vi "Add Ports Section.vi"(8 "error in":errorcluster, 11 "custom device ref":T1 format="%.0x") -> (0 "error out":errorcluster, 2 "ports ref":T1 format="%.0x", 3 "custom device ref out":T1 format="%.0x")   [LabVIEW 2020, in "ARINC 429 Scripting.lvlib"]
uses:
  ARINC 429 Scripting.lvlib
  <vilib>/NI VeriStand/Custom Device API/Custom Device Item Ref.ctl
  Ballard/Constants.vi
  <vilib>/NI VeriStand/Custom Device API/Custom Device API.lvlib
  Ballard/Ballard ARINC 429 Scripting.lvlib
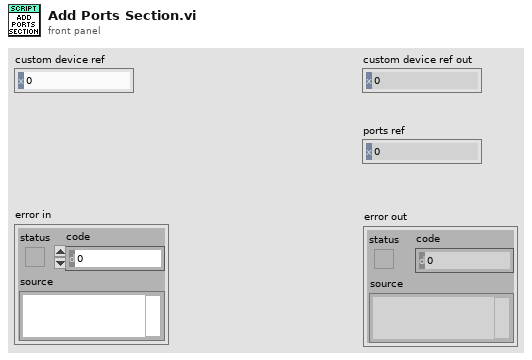
[diagram p1: front panel]
types:
  T1 = typedef "Custom Device API.lvlib/Custom Device Item Ref.ctl" = u64
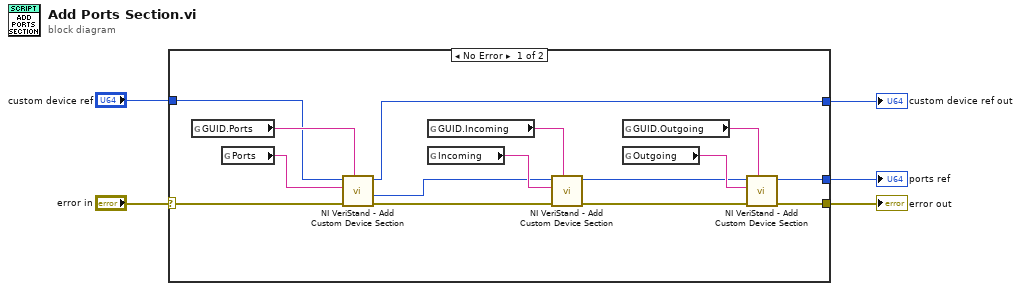
[diagram p0: block diagram]
diagram:
  n1 = case shown="No Error" "error in" {
    selector: "error in" -> [w18 w22]
    tunnel: "custom device ref" -> [w19 w21]
    tunnel: [w8 w22] -> w4
    tunnel: [w17 w21] -> w3
    tunnel: [w6 _] -> w1
    frame No Error {
      n2 = global read "Constants.vi" "GUID.Ports"() -> (w20:string)
      n3 = global read "Constants.vi" "Ports"() -> (w16:string)
      n4 = call <vilib>:"NI VeriStand - Add Custom Device Section.vi"("GUID (Default Section)"=w20, "error in (no error)"=w18, "Section Name"=w16, "Parent Ref in"=w19) -> ("error out"=w13:errorcluster, "Section Ptr"=w12:T1, "Parent Ref out"=w17:T1)  [unwired: 4 in, 1 out]
      n5 = global read "Constants.vi" "GUID.Incoming"() -> (w14:string)
      n6 = global read "Constants.vi" "Incoming"() -> (w15:string)
      n7 = call <vilib>:"NI VeriStand - Add Custom Device Section.vi"("GUID (Default Section)"=w14, "error in (no error)"=w13, "Section Name"=w15, "Parent Ref in"=w12) -> ("error out"=w9:errorcluster, "Parent Ref out"=w7:T1)  [unwired: 4 in, 2 out]
      n8 = global read "Constants.vi" "GUID.Outgoing"() -> (w10:string)
      n9 = global read "Constants.vi" "Outgoing"() -> (w11:string)
      n10 = call <vilib>:"NI VeriStand - Add Custom Device Section.vi"("GUID (Default Section)"=w10, "error in (no error)"=w9, "Section Name"=w11, "Parent Ref in"=w7) -> ("error out"=w8:errorcluster, "Parent Ref out"=w6:T1)  [unwired: 4 in, 2 out]
    }
    frame Error {
    }
  }
  "error out" <- w4
  "custom device ref out" <- w3
  "ports ref" <- w1
